vi "Check for Included Angle in Radians.vi"(5 "coerce output (F)":bool, 7 "output range (-pi to pi)":T1=enum."-pi to pi", 9 "right angle (rad)":dbl, 10 "target angle (rad)":dbl, 11 "left angle (rad)":dbl) -> (1 "in range?":bool, 2 "target angle out(rad)":dbl)   [LabVIEW 2017, in "NI_Robotics Utilities.lvlib"]
doc: "This VI is deprecated. Use <vi.lib>\\Analysis\\coordinate.llb\\Check for Included Angle.vi instead."
uses:
  <vilib>/robotics/Utilities/NI_Robotics Utilities.lvlib
  <vilib>/robotics/Utilities/Angle Range_Radians.ctl
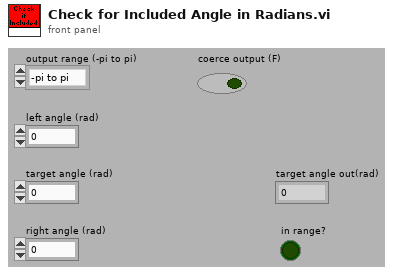
[diagram p1: front panel]
types:
  T1 = typedef "NI_Robotics Utilities.lvlib/Angle Range_Radians.ctl" = enum16{"none", "-pi to pi", "0 to 2*pi"}
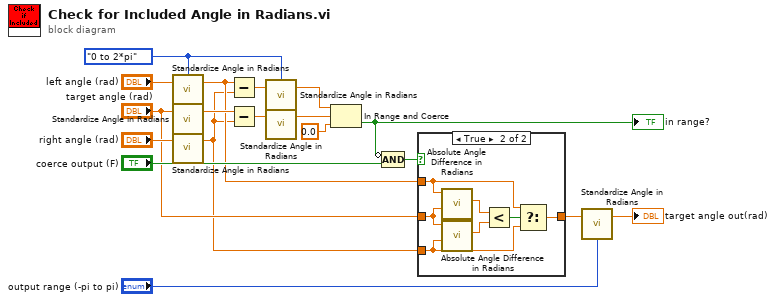
[diagram p0: block diagram]
diagram:
  w10 = Angle_Range_Radians."0 to 2*pi" ("range (-pi to pi)")
  n1 = call <vilib>:"Standardize Angle in Radians.vi"("angle in (rad)"="left angle (rad)", "range (-pi to pi)"=w10) -> ("angle out (rad)"=w6:dbl)  [unwired: 3 in]
  n2 = call <vilib>:"Standardize Angle in Radians.vi"("angle in (rad)"="target angle (rad)", "range (-pi to pi)"=w10) -> ("angle out (rad)"=w16:dbl)  [unwired: 3 in]
  n3 = call <vilib>:"Standardize Angle in Radians.vi"("angle in (rad)"="right angle (rad)", "range (-pi to pi)"=w10) -> ("angle out (rad)"=w4:dbl)  [unwired: 3 in]
  n4 = Subtract(x=w6, y=w4) -> (x-y=w14:dbl)
  n5 = Subtract(x=w16, y=w4) -> (x-y=w12:dbl)
  n6 = call <vilib>:"Standardize Angle in Radians.vi"("angle in (rad)"=w14, "range (-pi to pi)"=w10) -> ("angle out (rad)"=w13:dbl)  [unwired: 3 in]
  n7 = call <vilib>:"Standardize Angle in Radians.vi"("angle in (rad)"=w12, "range (-pi to pi)"=w10) -> ("angle out (rad)"=w11:dbl)  [unwired: 3 in]
  n8 = In Range and Coerce(upper limit=w13, x=w11, lower limit=0.0) -> (In Range?=w8:bool)  [unwired: 1 out]
  "in range?" <- w8
  n9 = Compound Arithmetic op=AND(invert w8, "coerce output (F)") -> (w9:bool)
  n10 = case shown="True" w9 {
    tunnel: w6 -> [_ w22]
    tunnel: "target angle (rad)" -> [w19 w26]
    tunnel: w4 -> [_ w21]
    tunnel: [w19 w20] -> w3
    frame False {
    }
    frame True {
      n11 = call <vilib>:"Absolute Angle Difference in Radians.vi"("angle 2 (rad)"=w26, "angle 1 (rad)"=w22) -> ("|angle 1 - angle 2| (rad)"=w25:dbl)  [unwired: 9 in]
      n12 = call <vilib>:"Absolute Angle Difference in Radians.vi"("angle 2 (rad)"=w21, "angle 1 (rad)"=w26) -> ("|angle 1 - angle 2| (rad)"=w24:dbl)  [unwired: 9 in]
      n13 = Less?(x=w25, y=w24) -> (x < y?=w23:bool)
      n14 = Select(t=w22, s=w23, f=w21) -> (s? t:f=w20:dbl)
    }
  }
  n15 = call <vilib>:"Standardize Angle in Radians.vi"("angle in (rad)"=w3, "range (-pi to pi)"="output range (-pi to pi)") -> ("angle out (rad)"=→"target angle out(rad)":dbl)  [unwired: 3 in]
